vi "22_2.vi"() -> ()   [LabVIEW 2020]
panel:
  out "Player 1 Wins":bool=TRUE
  out "Score":i32=31835
  in  "Switch":bool
  in  "Input":string="Player 1:\n28\n13\n25\n16\n38\n3\n14\n6\n29\n2\n47\n20\n35\n43\n30\n39\n21\n42\n50\n48\n23\n11\n34\n24\n41\n\nPlayer 2:\n27\n37\n9\n10\n17\n31\n19\n33\n40\n12\n32\n1\n18\n36\n49\n46\n26\n4\n45\n8\n15\n5\n44\n22\n7"
  in  "Input Test":string="Player 1:\n9\n2\n6\n3\n1\n\nPlayer 2:\n5\n8\n4\n7\n10"
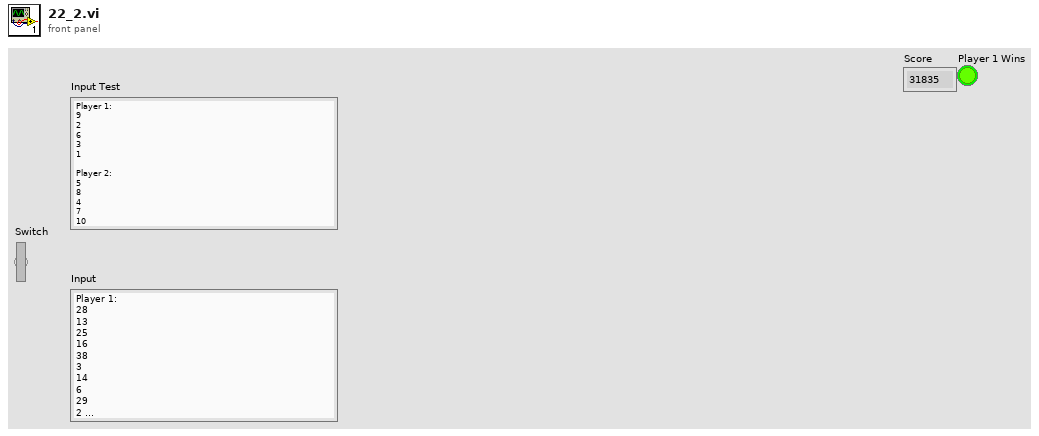
[diagram p1: front panel]
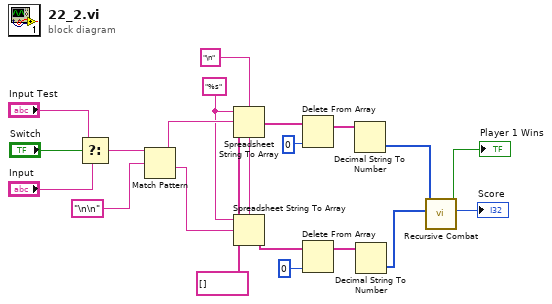
[diagram p0: block diagram]
diagram:
  w14 = string[] []
  w11 = "\n"
  w13 = "%s"
  n1 = Select(t="Input Test", s="Switch", f="Input") -> (s? t:f=w17:string)
  n2 = Match Pattern(string=w17, regular expression="\n\n") -> (before substring=w15:string, after substring=w12:string)  [unwired: 1 in, 2 out]
  n3 = Spreadsheet String To Array(delimiter (Tab)=w11, format string=w13, spreadsheet string=w15, array type (2D Dbl)=w14) -> (array=w10:string[])
  n4 = Spreadsheet String To Array(delimiter (Tab)=w11, format string=w13, spreadsheet string=w12, array type (2D Dbl)=w14) -> (array=w9:string[])
  n5 = Delete From Array(array=w10, index=0) -> (array with subset deleted=w7:string[])  [unwired: 1 in, 1 out]
  n6 = Delete From Array(array=w9, index=0) -> (array with subset deleted=w6:string[])  [unwired: 1 in, 1 out]
  n7 = Decimal String To Number(string=w7) -> (number=w2:i32[])  [unwired: 2 in, 1 out]
  n8 = Decimal String To Number(string=w6) -> (number=w5:i32[])  [unwired: 2 in, 1 out]
  n9 = call "Recursive Combat.vi"("Player 2 Deck"=w5, "Player 1 Deck"=w2) -> ("Score"=→"Score":i32, "Player 1 wins"=→"Player 1 Wins":bool)  [unwired: 8 in]
